vi "DRC91ReadTemp.vi"(0 "VISA Rsrc":refnum<visa-resource-name>="GPIB0::12::INSTR", 5 "Activées":bool[](array[boolean])=[TRUE, FALSE] caption="Entrés Activées", 11 "error in":errorcluster) -> (4 "Données":dbl[](array[numeric]), 6 "Units":string[](array[string]), 15 "error out":errorcluster)   [LabVIEW 2010]
doc: "This VI querys the instrument for an inputs sensor reading in Celsius, Kelvin, and Sensor Units."
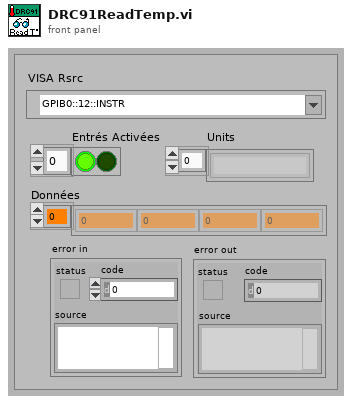
[diagram p1: front panel]
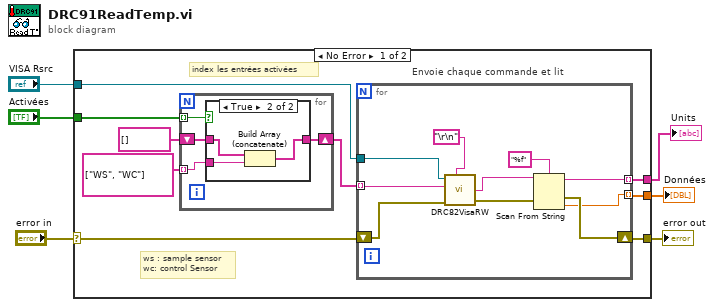
[diagram p0: block diagram]
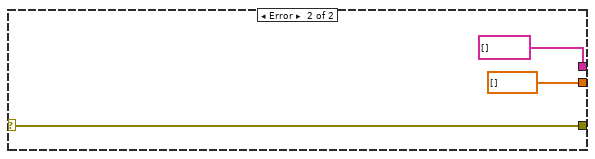
[diagram p3: hidden frame]
diagram:
  n1 = case shown="No Error" "error in" {
    selector: "error in" -> [w12 w36]
    tunnel: [w15 w36] -> w6
    tunnel: "VISA Rsrc" -> [w14 _]
    tunnel: [w13 dbl[] []] -> w4
    tunnel: "Activées" -> [w10 _]
    tunnel: [w7 string[] []] -> w1
    frame No Error {
      # "ws : sample sensor\nwc: control Sensor"
      # "index les entrées activées"
      # "Envoie chaque commande et lit"
      n2 = for {
        tunnel: string[] ["WS", "WC"] -> [w18] mode=indexing
        tunnel: w10 -> [w19] mode=indexing
        shift-right: [w17] -> w8
        shift-left: string[] [] -> [w16]
        n3 = case shown="True" w19 {
          tunnel: w18 -> [_ w22]
          tunnel: [w20 w23] -> w17
          tunnel: w16 -> [w20 w21]
          frame False {
          }
          frame True {
            n4 = Build Array (concatenate)(w21, w22) -> (w23:string[])
          }
        }
      }
      n5 = for {
        tunnel: w8 -> [w33] mode=indexing
        shift-right: [w27] -> w15
        shift-left: w12 -> [w31]
        tunnel: w14 -> [w32]
        tunnel: [w26] -> w13 mode=indexing
        tunnel: [w24] -> w7 mode=indexing
        n6 = call <userlib>:"DRC82VisaRW.vi"("error in (no error)"=w31, "EOS (Aucun)"="\r\n", "ChaineCom"=w33, "VISA Rsrc"=w32) -> ("error out"=w28:errorcluster, "ChaineRep"=w29:string)  [unwired: 3 in, 2 out]
        n7 = Scan From String(format string="%f", input string=w29, error in=w28) -> (remaining string=w24:string, error out=w27:errorcluster, output 1=w26:dbl)  [unwired: 2 in, 1 out]
      }
    }
    frame Error {
    }
  }
  "error out" <- w6
  "Données" <- w4
  "Units" <- w1
